vi "getUpdateDefaultAmountStatement.vi"(8 "error in (no error)":errorcluster, 11 "Category in":refnum<class "Category.lvclass">) -> (0 "error out":errorcluster, 2 "Update Statement":string, 3 "Category out":refnum<class "Category.lvclass">)   [LabVIEW 2018, in "Category.lvclass"]
uses:
  Category.lvclass
  Category.lvclass/Category.ctl
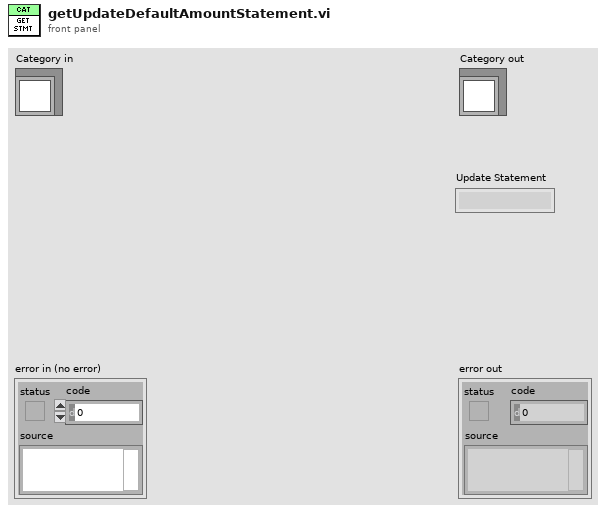
[diagram p1: front panel]
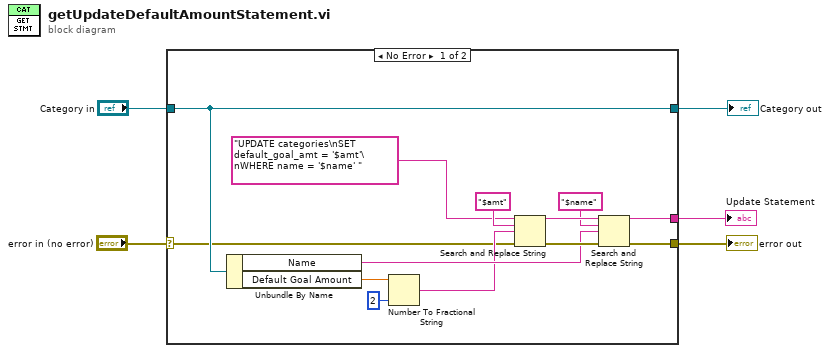
[diagram p0: block diagram]
diagram:
  n1 = case shown="No Error" "error in (no error)" {
    selector: "error in (no error)" -> [w8 w20]
    tunnel: [w7 w20] -> w4
    tunnel: [w18 w19] -> w2
    tunnel: "Category in" -> [w18 w19]
    tunnel: [w6 _] -> w1
    frame No Error {
      n2 = Unbundle By Name(w18) -> ("Name"=w10:string, "Default Goal Amount"=w16:dbl)
      n3 = Number To Fractional String(number=w16, precision (6)=i16 2) -> (F-format string=w9:string)  [unwired: 2 in]
      n4 = Search and Replace String(input string="UPDATE categories\nSET default_goal_amt = '$amt'\nWHERE name = '$name' ", search string="$amt", replace string=w9, error in=w8) -> (result string=w14:string, error out=w15:errorcluster)  [unwired: 4 in, 2 out]
      n5 = Search and Replace String(input string=w14, search string="$name", replace string=w10, error in=w15) -> (result string=w6:string, error out=w7:errorcluster)  [unwired: 4 in, 2 out]
    }
    frame Error {
    }
  }
  "error out" <- w4
  "Category out" <- w2
  "Update Statement" <- w1
